vi "PRIME Detector Send START.vi"(8 "error in (no error)":errorcluster, 10 "Exposure Time":dbl, 11 "connection ID":refnum<k5>[](array[refnum])) -> (0 "error out":errorcluster, 3 "connection ID out":refnum<k5>[](array[refnum]))   [LabVIEW 2021, in "PRIME Detector.lvclass"]
uses:
  PRIME Detector.lvclass
panel:
  out "Status":string
  out "Responses":string[](array[string])
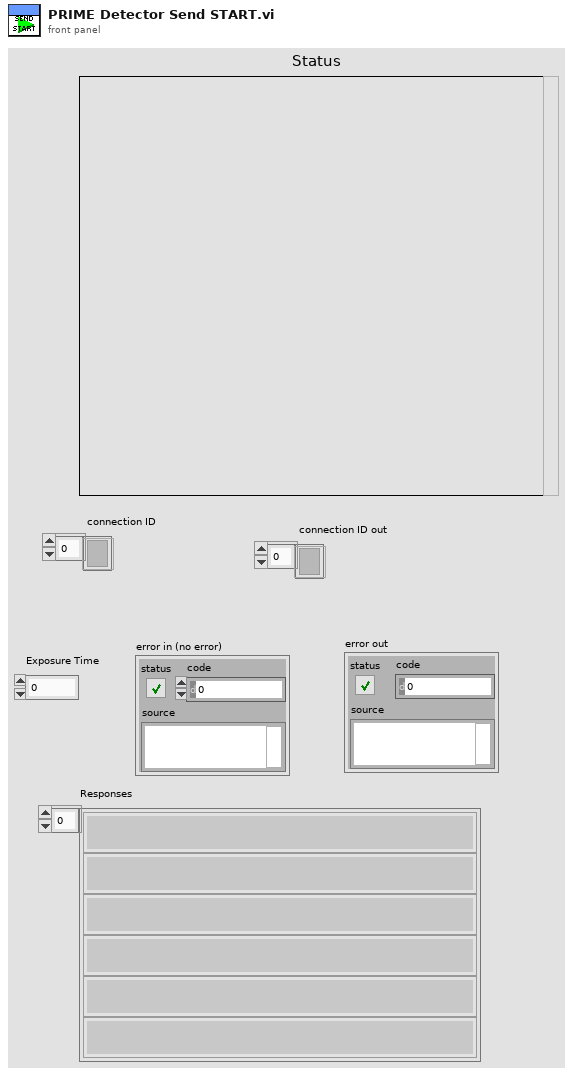
[diagram p1: front panel]
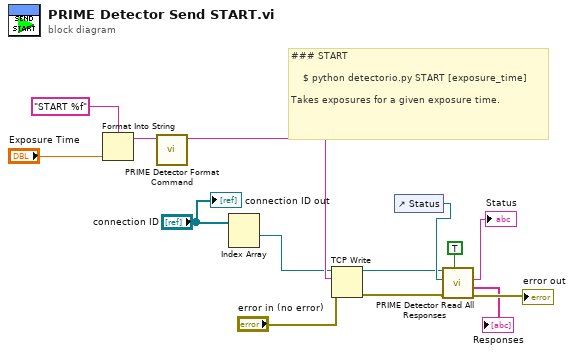
[diagram p0: block diagram]
diagram:
  # "### START\n\n    $ python detectorio.py START [exposure_time]\n\nTakes exposures for a given exposure time."
  n1 = Format Into String(format string="START %f" ("Command"), "Exposure Time") -> (resulting string=w2:string)  [unwired: 2 in, 1 out]
  n2 = call "PRIME Detector Format Command.vi"("Command"=w2) -> ("TCP String"=w14:string)  [unwired: 10 in]
  n3 = Index Array(array="connection ID") -> (element #1=w6:refnum<k5>)  [unwired: 2 in, 1 out]
  n4 = TCP Write(connection ID=w6, data in=w14, error in (no error)="error in (no error)") -> (connection ID out=w4:refnum<k5>, error out=w12:errorcluster)  [unwired: 1 in, 1 out]
  n5 = control-ref of="Status"() -> (w7:refnum<vi>)
  n6 = call "PRIME Detector Read All Responses.vi"("Log"=TRUE, "error in"=w12, "Str Ref"=w7, "connection ID"=w4) -> ("error out"=→"error out":errorcluster, "Responses"=→"Responses":string[], "Status Response"=→"Status":string)  [unwired: 4 in, 1 out]
  "connection ID out" <- "connection ID"
